vi "Do Get Object Help.vi"(8 "error in (no error)":errorcluster, 10 "get_object_help Argument":T2, 11 "Data Cluster in":T1) -> (0 "error out":errorcluster, 2 "help_string":string, 3 "Data Cluster out":T1)   [LabVIEW 2025, in "Scripting Server.lvlib"]
uses:
  Scripting Server.lvlib
  get_object_help Argument--cluster.ctl
  get_object_help (Reply Payload)--cluster.ctl
  Module Data--cluster.ctl
panel:
  out "help tag":string
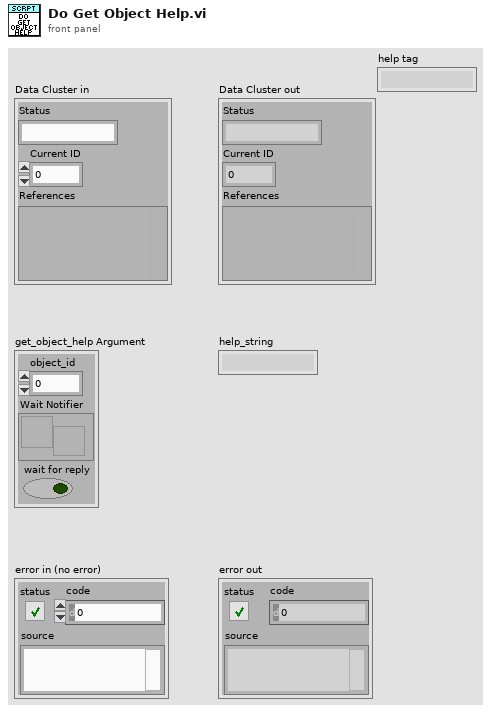
[diagram p1: front panel]
types:
  T1 = typedef "Scripting Server.lvlib/Module Data--cluster.ctl" = cluster{"Status":string, "Current ID":i32, "References":variant}
  T2 = typedef "Scripting Server.lvlib/get_object_help Argument--cluster.ctl" = cluster{"object_id":i32, "Wait Notifier":refnum<notifier>, "wait for reply":bool}
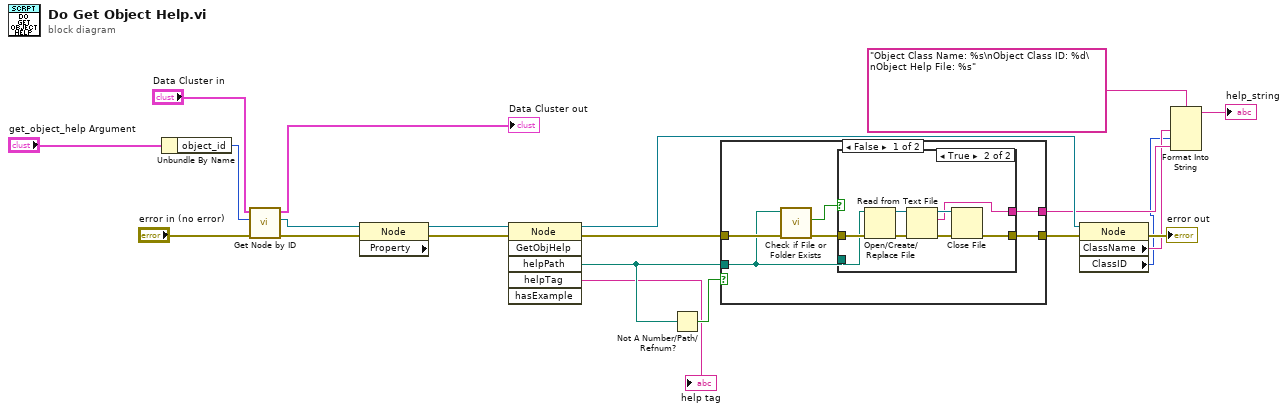
[diagram p0: block diagram]
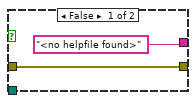
[diagram p2: hidden frame]
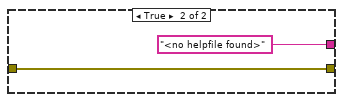
[diagram p3: hidden frame]
diagram:
  n1 = Unbundle By Name("get_object_help Argument") -> ("object_id"=w16:i32)
  n2 = call "Get Node by ID.vi"("error in (no error)"="error in (no error)", "ID"=w16, "Data Cluster in"="Data Cluster in") -> ("error out"=w19:errorcluster, "specific class reference"=w2:refnum<vi>, "Data Cluster out"=→"Data Cluster out":T1)  [unwired: 6 in]
  n3 = property class="Node" props=[](reference=w2, error in=w19) -> (reference out=w1:refnum<vi>, error out=w3:errorcluster)  [unwired: 1 out]
  n4 = invoke class="Node" method="GetObjHelp"(reference=w1, error in=w3) -> (reference out=w13:refnum<vi>, error out=w14:errorcluster, "helpPath"=w10:path, "helpTag"=→"help tag":string)  [unwired: 4 in, 2 out]
  n5 = Not A Number/Path/Refnum?(number/path/refnum=w10) -> (NaN/Path/Refnum?=w11:bool)
  n6 = case shown="False" w11 {
    tunnel: w14 -> [w27 w39]
    tunnel: [w26 w39] -> w12
    tunnel: w10 -> [w23 _]
    tunnel: [w25 "<no helpfile found>"] -> w7
    frame False {
      n7 = call <vilib>:"Check if File or Folder Exists.vi"("error in (no error)"=w27, "path"=w23) -> ("error out"=w24:errorcluster, "file or folder exists?"=w22:bool)  [unwired: 7 in, 1 out]
      n8 = case shown="True" w22 {
        tunnel: [w29 w35] -> w26
        tunnel: ["<no helpfile found>" w32] -> w25
        tunnel: w24 -> [w29 w31]
        tunnel: w23 -> [_ w30]
        frame False {
        }
        frame True {
          n9 = Open/Create/Replace File(file path (use dialog)=w30, error in=w31) -> (refnum out=w34:refnum<file>, error out=w37:errorcluster)  [unwired: 4 in, 1 out]
          n10 = Read from Text File(file (use dialog)=w34, error in=w37) -> (refnum out=w33:refnum<file>, text=w32:string, error out=w36:errorcluster)  [unwired: 2 in, 1 out]
          n11 = Close File(refnum=w33, error in=w36) -> (error out=w35:errorcluster)  [unwired: 1 out]
        }
      }
    }
    frame True {
    }
  }
  n12 = property class="Node"(reference=w13, error in=w12) -> (error out=→"error out":errorcluster, "ClassName"=w6:string, "ClassID"=w5:u32)  [unwired: 1 out]
  n13 = Format Into String(format string="Object Class Name: %s\nObject Class ID: %d\nObject Help File: %s", w6, w5, w7) -> (resulting string=→"help_string":string)  [unwired: 2 in, 1 out]
